vi "feedback.vi"() -> ()   [LabVIEW 2014]
uses:
  <vilib>/FTP/NI_FTP.lvlib
panel:
  in  "확인 버튼 2":bool
  in  "확인 버튼":bool
  in  "닫기":bool
  in  "Subject":string="받는사람" caption="제목"
  in  "Message":string="제목을 입력해 주세요." caption="메시지"
  # "메시지전송"
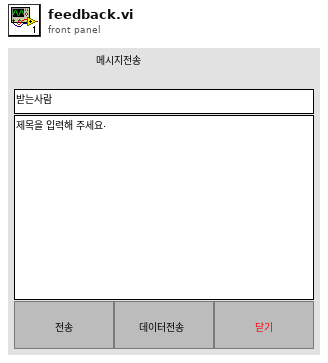
[diagram p1: front panel]
types:
  T1 = typedef "NI_FTP.lvlib/FTP Session.ctl" = refnum<k5>
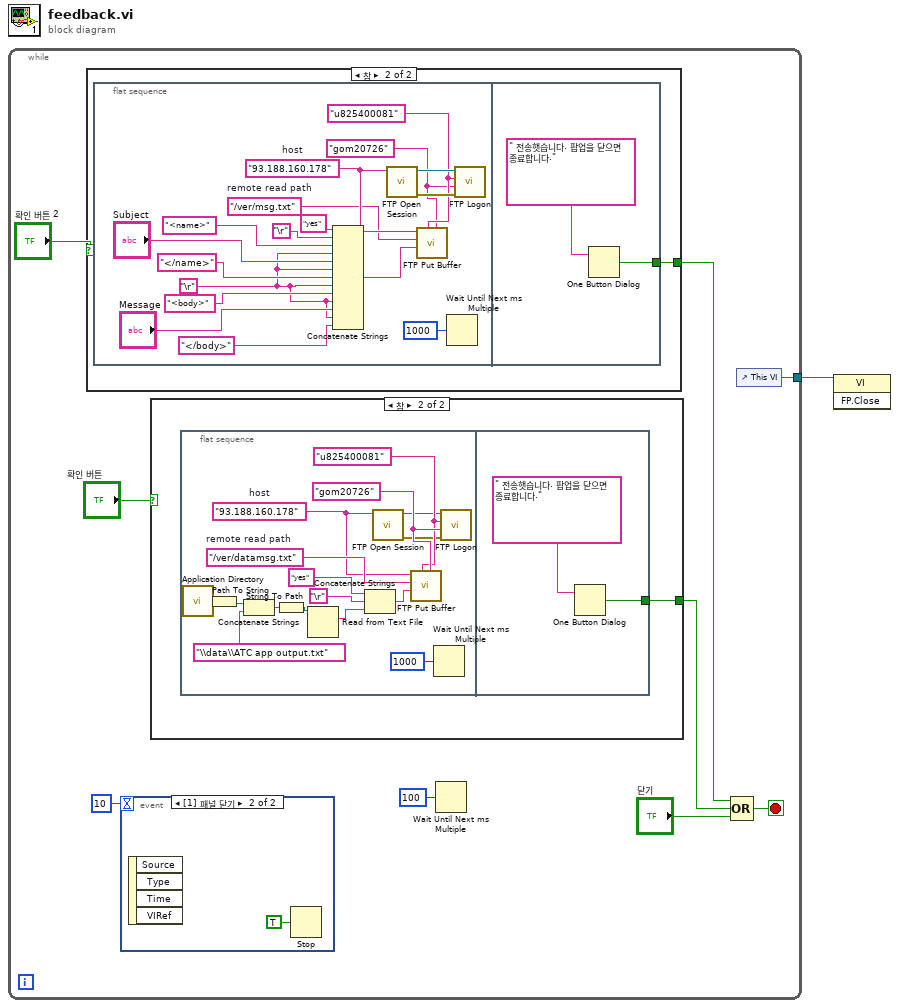
[diagram p0: block diagram]
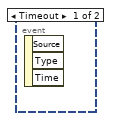
[diagram p2: hidden frame]
diagram:
  n1 = while {
    tunnel: [w10] -> w1
    stop <- w7 stop-if-true
    n2 = case shown="참" "확인 버튼 2" {
      tunnel: [_ w31] -> w4
      frame False {
      }
      frame True {
        n3 = flat-sequence {
          tunnel: [w49] -> w31
          frame #0 {
            w36 = "\r"
            w45 = "gom20726"
            w46 = "u825400081"
            w41 = "/ver/msg.txt"  # remote read path
            w44 = "93.188.160.178"  # host
            n4 = Concatenate Strings("yes", "\r", "<name>" ("문자열"), w36, "Subject", w36, "</name>" ("문자열"), w36, "<body>" ("문자열"), w36, "Message", w36, "</body>" ("문자열")) -> (w42:string)
            n5 = call <vilib>:"FTP Open Session.vi"("address"=w44) -> ("error out"=w47:errorcluster, "ftp session"=w48:T1)  [unwired: 7 in, 2 out]
            n6 = call <vilib>:"FTP Put Buffer.vi"("password"=w45, "user"=w46, "data"=w42, "remote path"=w41, "host"=w44) -> ()  [unwired: 5 in, 2 out]
            n7 = Wait Until Next ms Multiple(millisecond multiple=u32 1000 ("ms 배수")) -> ()  [unwired: 1 out]
            n8 = call <vilib>:"FTP Logon.vi"("error in (no error)"=w47, "password"=w45, "user"=w46, "ftp session"=w48) -> ()  [unwired: 4 in, 4 out]
          }
          frame #1 {
            n9 = One Button Dialog(message=" 전송햇습니다. 팝업을 닫으면 종료합니다." ("메시지")) -> (true=w49:bool)  [unwired: 1 in]
          }
        }
      }
    }
    n10 = event shown="[1] 패널 닫기" {
      selector: _ -> [_ _]
      dyn-events: _ -> [_ _]
      timeout: 10 -> [_ _]
      event Timeout {
        n11 = event-data() -> ()  [unwired: 1 in, 3 out]
      }
      event Panel Close {
        n12 = event-data() -> ()  [unwired: 1 in, 4 out]
        n13 = Stop(stop? (T)=TRUE ("정지? (참)")) -> ()
      }
    }
    n14 = case shown="참" "확인 버튼" {
      tunnel: [_ w12] -> w5
      frame False {
      }
      frame True {
        n15 = flat-sequence {
          tunnel: [w29] -> w12
          frame #0 {
            w26 = "gom20726"
            w25 = "u825400081"
            w28 = "/ver/datamsg.txt"  # remote read path
            w27 = "93.188.160.178"  # host
            n16 = call <vilib>:"Application Directory.vi"() -> ("Application Directory"=w22:path)
            n17 = Path To String(path=w22) -> (string=w20:string)
            n18 = Concatenate Strings(w20, "\\data\\ATC app output.txt" ("문자열")) -> (w19:string)
            n19 = String To Path(string=w19) -> (path=w18:path)
            n20 = Read from Text File(file (use dialog)=w18) -> (text=w15:string)  [unwired: 3 in, 3 out]
            n21 = Concatenate Strings("yes", "\r", w15) -> (w13:string)
            n22 = call <vilib>:"FTP Open Session.vi"("address"=w27) -> ("error out"=w24:errorcluster, "ftp session"=w23:T1)  [unwired: 7 in, 2 out]
            n23 = call <vilib>:"FTP Put Buffer.vi"("password"=w26, "user"=w25, "data"=w13, "remote path"=w28, "host"=w27) -> ()  [unwired: 5 in, 2 out]
            n24 = Wait Until Next ms Multiple(millisecond multiple=u32 1000 ("ms 배수")) -> ()  [unwired: 1 out]
            n25 = call <vilib>:"FTP Logon.vi"("error in (no error)"=w24, "password"=w26, "user"=w25, "ftp session"=w23) -> ()  [unwired: 4 in, 4 out]
          }
          frame #1 {
            n26 = One Button Dialog(message=" 전송햇습니다. 팝업을 닫으면 종료합니다." ("메시지")) -> (true=w29:bool)  [unwired: 1 in]
          }
        }
      }
    }
    n27 = Wait Until Next ms Multiple(millisecond multiple=u32 100 ("ms 배수")) -> ()  [unwired: 1 out]
    n28 = Compound Arithmetic op=OR(w4, w5, "닫기") -> (w7:bool)
    n29 = control-ref of="This VI"() -> (w10:refnum<vi>)
  }
  n30 = invoke class="VI" method="FP.Close"(reference=w1) -> ()  [unwired: 2 in, 3 out]
